vi "读取当天数据库信息.vi"() -> (3 "Results":string[][][](array[string]))   [LabVIEW 2017]
uses:
  Sqlite/CBB/ReadAllData.vi
  Sqlite/SQLite.lvlib
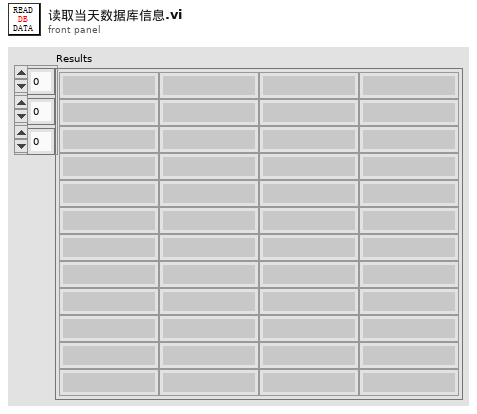
[diagram p1: front panel]
types:
  T1 = cluster{"设备明细":cluster{"table":string, "column":string[]}, "ER":cluster{"table":string, "column":string[]}}
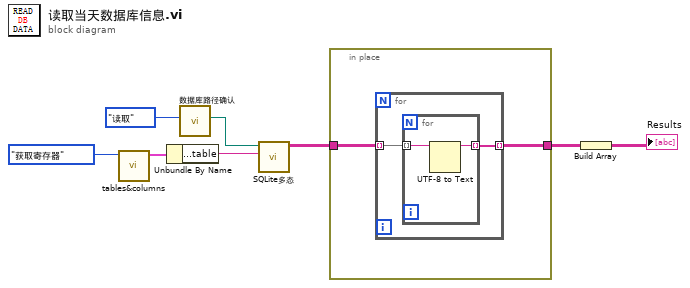
[diagram p0: block diagram]
diagram:
  n1 = call "tables&columns.vi"("选项"=enum16{"初始化", "获取寄存器"}."获取寄存器") -> ("Tables&columns"=w4:T1)  [unwired: 9 in, 1 out]
  n2 = Unbundle By Name(w4) -> ("设备明细.table"=w3:string)
  n3 = call "数据库路径确认.vi"("选项"=enum16{"初始化", "读取"}."读取") -> ("数据库路径"=w6:path)  [unwired: 10 in]
  n4 = call-poly "SQLite多态.vi"("Table Name"=w3, "DbPath"=w6) -> ("Results"=w7:string[][])  [unwired: 4 in, 5 out]
  n5 = in-place {
    in-place-border: [w10] -> w2
    in-place-border: w7 -> [w9]
    n6 = for {
      tunnel: w9 -> [w12] mode=indexing
      tunnel: [w11] -> w10 mode=indexing
      n7 = for {
        tunnel: w12 -> [w14] mode=indexing
        tunnel: [w13] -> w11 mode=indexing
        n8 = UTF-8 to Text(11:w14) -> (3:w13:string)  [unwired: 2 in, 1 out]
      }
    }
  }
  n9 = Build Array(w2) -> (→"Results":string[][][])
